vi "As Ref.vi"(11 "Headers in":refnum<class "Headers.lvclass">) -> (2 "ref":u64)   [LabVIEW 2020, in "reqwest.lvlib" / "Headers.lvclass"]
uses:
  Headers.lvclass
  Headers.lvclass/Headers.ctl
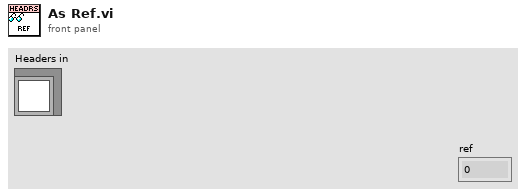
[diagram p1: front panel]
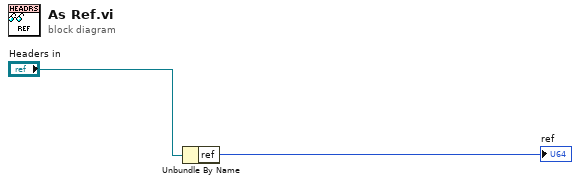
[diagram p0: block diagram]
diagram:
  n1 = Unbundle By Name("Headers in") -> ("ref"=→"ref":u64)
